vi "UTILITY Append Byte To Read TCP.vi"(8 "Error In":errorcluster, 11 "Input String":string) -> (0 "Error Out":errorcluster, 3 "Output String":string)   [LabVIEW 2016]
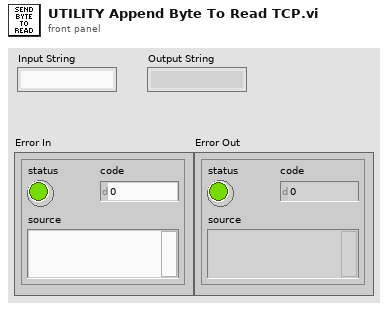
[diagram p1: front panel]
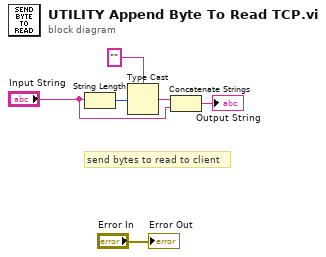
[diagram p0: block diagram]
diagram:
  # "send bytes to read to client"
  n1 = String Length(string="Input String") -> (length=w6:i32)
  n2 = Type Cast(type="", x=w6) -> (*(type *) &x=w5:string)
  n3 = Concatenate Strings(w5, "Input String") -> (→"Output String":string)
  "Error Out" <- "Error In"
